vi "Vision Processing.vi"(4 "error in (no error)":errorcluster, 6 "CameraDevRef":T1) -> ()   [LabVIEW 2011]
uses:
  <vilib>/Rock Robotics/WPI/Camera/WPI_CameraDevRef.ctl
  Robot Global Data.vi
  <vilib>/vision/NI_Vision_Development_Module.lvlib
panel:
  in  "Scale":dbl=0.85
  in  "Minimum Power":dbl=0.2
  out "Aspect Ratio":dbl[](array[numeric])
  out "Offset":dbl
  in  "Max Distance for 1 hoop":dbl=8.0
  out "Raw Turret":dbl
  in  "Run Calculations":bool=TRUE
  out "Target X Coord":dbl
  out "Target Distance":dbl
  out "Target Y Coord":dbl
  out "Distance Array":dbl[](array[numeric])
  in  "Dead Band":dbl=0.1
  out "Number of Rectangles Visible":dbl
  out "Y Position Array":dbl[](array[numeric])
  out "X Position Array":dbl[](array[numeric])
  in  "View":bool
  out "Target Info":T2(array[cluster])
  in  "Area Size Limit":i32=444
  in  "Particle Count Limit":i32=8
  in  "Score Limits":T3={"Rect Coverage"=76.0, "Aspect Ratio"=40.0, "X Edge Strength"=40.0, "Y Edge Strength"=60.0}
  in  "Processing":enum32{"Color", "Intensity", "Intensity Open"}(tab)=enum."Intensity"
  in  "Luminance":i32=255
  in  "Saturation":i32=255
  in  "Hue":i32(knob)=65 scale=0.0..255.0
  in  "Margins":cluster{"Hue":i32, "Sat":i32, "Lum":i32}={"Hue"=20, "Sat"=27, "Lum"=30} {"Sat" scale=0.0..40.0; "Lum" scale=0.0..40.0; "Hue" scale=0.0..40.0}
  in  "Range":cluster{"Lower value":sgl, "Upper value":sgl}={"Lower value"=107.17391, "Upper value"=255.0} {"Lower value" scale=0.0..255.0; "Upper value" scale=0.0..255.0}
  in  "Range":cluster{"Lower value":sgl, "Upper value":sgl}={"Lower value"=123.804344, "Upper value"=255.0} {"Lower value" scale=0.0..255.0; "Upper value" scale=0.0..255.0}
  in  "View":bool
  out "Processed Image":T4(plugin-control)
  out "Original Image":T4(plugin-control)
  # "Instructions:\nProcessing the reflective tape that is illuminated by a ring light can be based\non color or light intensity.\nParticles within the image are scored by rectangle coverage, aspect ratio, and\nfor being hollow with a bold edge. A particle is considered a target if all scores\nare above the score limits. Particles can be annotated -- surrounded by\na rectangle and scores drawn to the left .\nTo control the number of particles being scored, use the count limit and the size\nlimit."
  # "(in)"
  # "To debug, Enable using the View button.\nFor color processing, you can click in the image to select the color for processing."
  # "Enable by clicking the View button.\nGreen scores are above the limit, orange are below. Inner/outer rect\nindicates all passed."
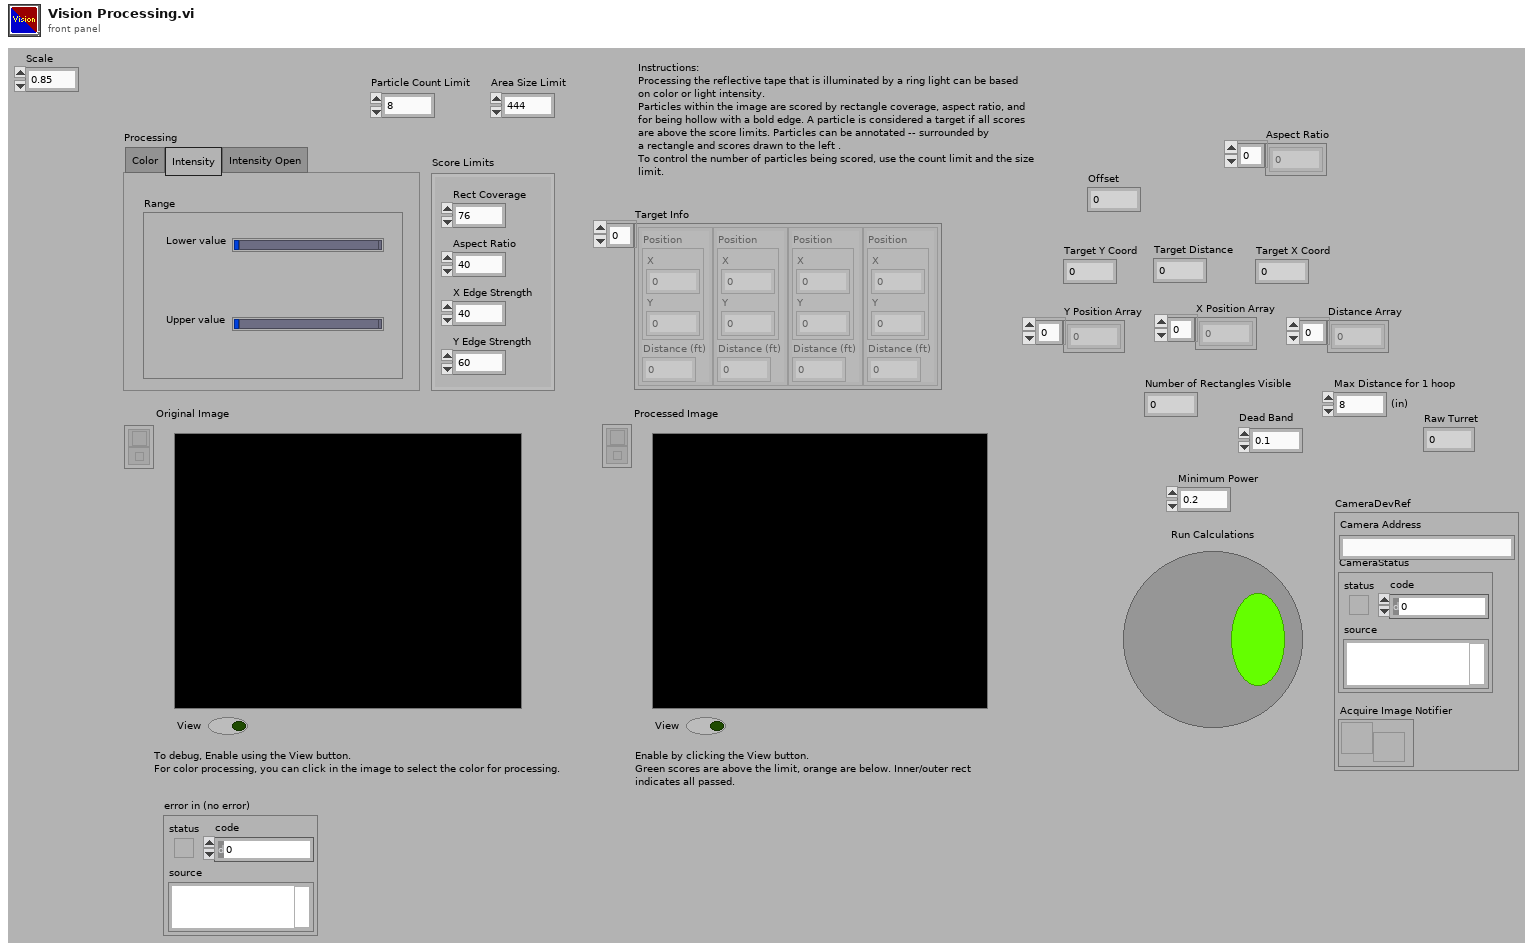
[diagram p1: front panel]
types:
  T1 = typedef "WPI_CameraDevRef.ctl" = cluster{"Camera Address":string, "CameraStatus":errorcluster, "Acquire Image Notifier":refnum<notifier>}
  T2 = cluster{"Position":cluster{"X":dbl, "Y":dbl}, "Distance (ft)":dbl}[]
  T3 = cluster{"Rect Coverage":dbl, "Aspect Ratio":dbl, "X Edge Strength":dbl, "Y Edge Strength":dbl}
  T4 = typedef "IMAQ Image.ctl" = refnum<image>
  T5 = typedef "Image Type" = u32
  T6 = enum32{"AutoM", "Close", "Dilate", "Erode", "Gradient", "Gradient out", "Gradient in", "Hit miss", "Open", "PClose", "POpen", "Thick", "Thin"}
  T7 = typedef "WPI_CameraImageSize.ctl" = enum16{"640x480", "320x240", "160x120"}
  T8 = cluster{"fps":i32, "compression":i32, "Image Size":T7}
  T9 = cluster{cluster{"Left":dbl, "Top":dbl, "Right":dbl, "Bottom":dbl}, dbl[]}[]
  T10 = cluster{"Left":dbl, "Top":dbl, "Right":dbl, "Bottom":dbl}
  T11 = cluster{"Target Center (-1 to 1)":cluster{"X":dbl, "Y":dbl}, "Distance (ft)":dbl}
  T12 = cluster{"Target Center (-1 to 1)":cluster{"X":dbl, "Y":dbl}, "Distance (ft)":dbl}[]
  T13 = typedef "WPI_JoystickDevRef.ctl" = cluster{"Device":T14}
  T14 = typedef "WPI_JoystickDeviceEnum.ctl" = enum16{"USB 1", "USB 2", "USB 3", "USB 4", "Kinect 1", "Kinect 2"}
  T15 = typedef "WPI_JoystickButtonState.ctl" = cluster{"Button 1":bool, "Button 2":bool, "Button 3":bool, "Button 4":bool, "Button 5":bool, "Button 6":bool, "Button 7":bool, "Button 8":bool, "Button 9":bool, "Button 10":bool, "Button 11":bool, "Button 12":bool}
  T16 = cluster{"axis 1 (x)":dbl, "axis 2 (y)":dbl, "axis 3 (throttle)":dbl, "axis 4":dbl, "axis 5":dbl, "axis 6":dbl}
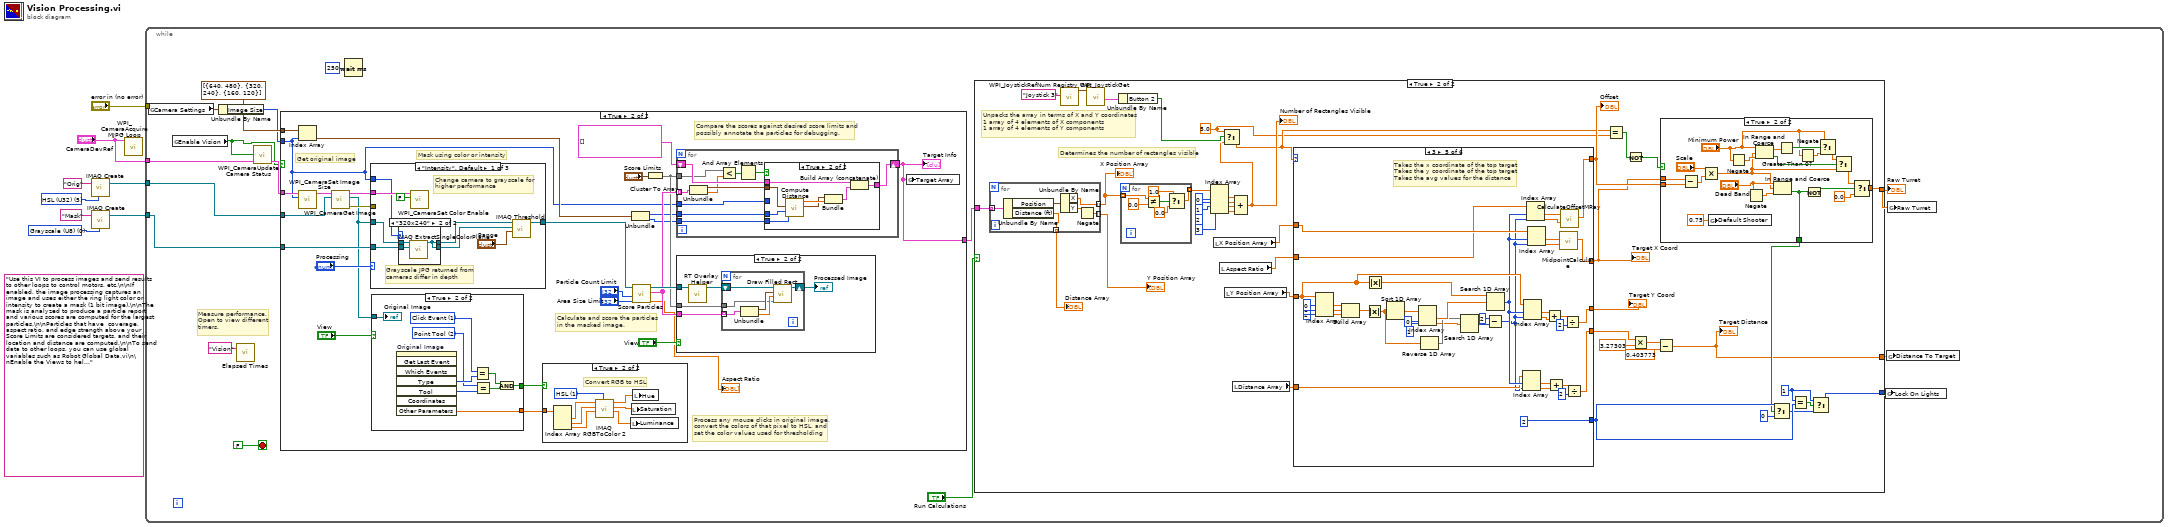
[diagram p0: block diagram]
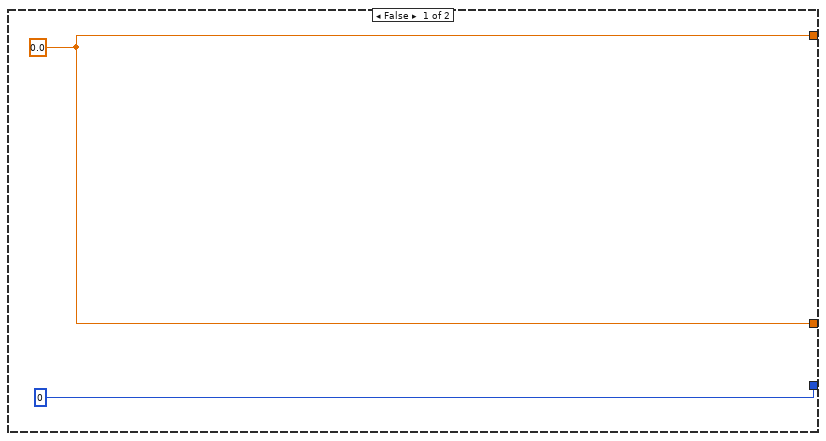
[diagram p2: hidden frame]
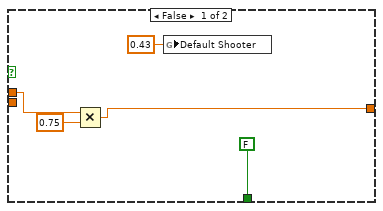
[diagram p3: hidden frame]
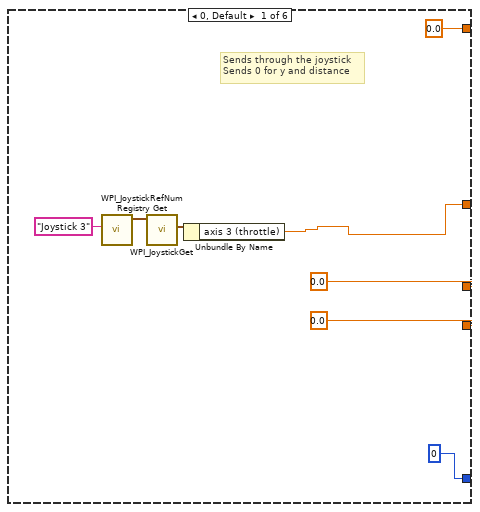
[diagram p4: hidden frame]
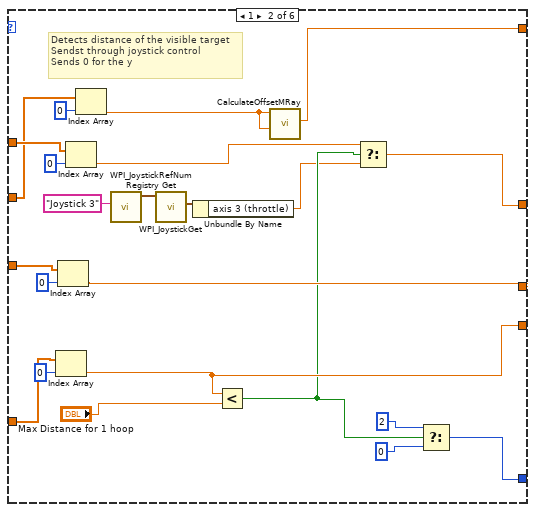
[diagram p5: hidden frame]
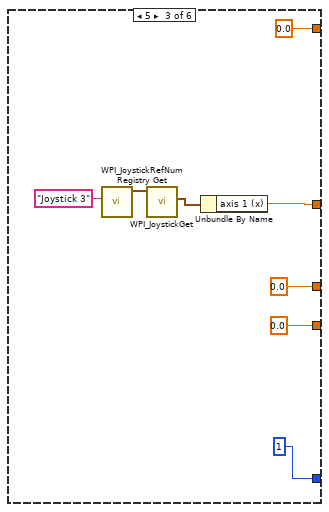
[diagram p6: hidden frame]
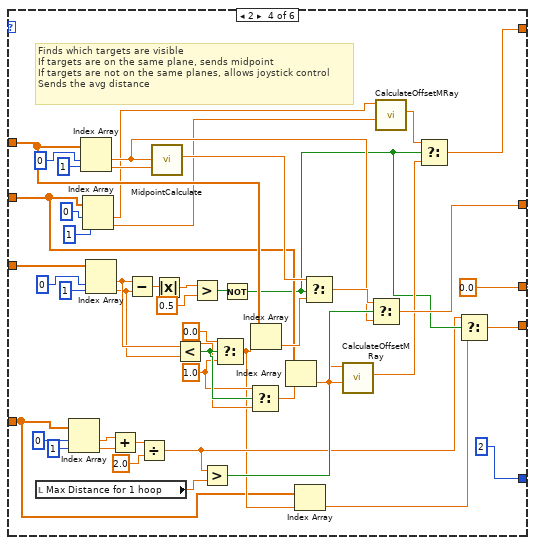
[diagram p7: hidden frame]
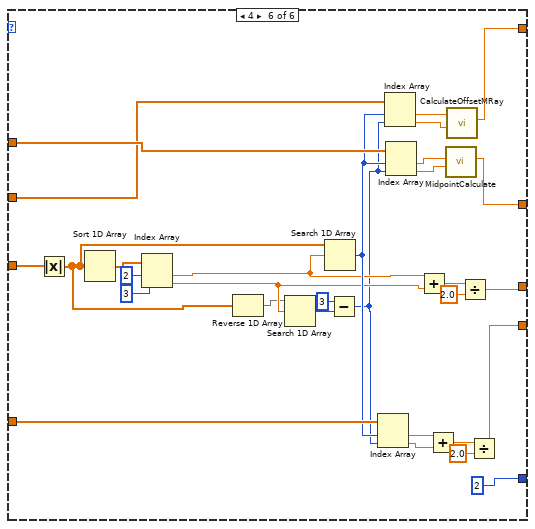
[diagram p8: hidden frame]
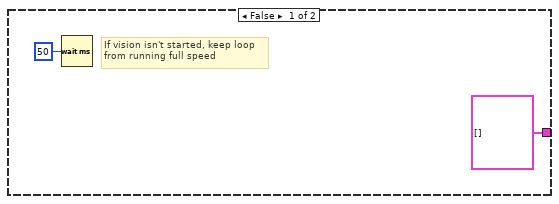
[diagram p9: hidden frame]
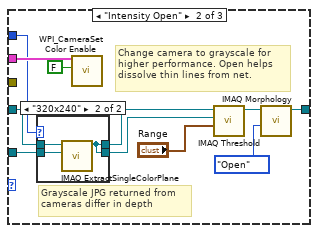
[diagram p12: hidden frame]
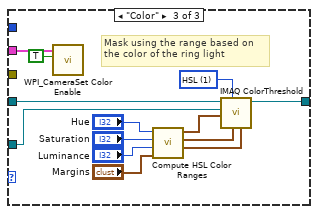
[diagram p14: hidden frame]
diagram:
  w3 = T5 0 items=["Grayscale (U8)", "Grayscale (I16)", "Grayscale (SGL)", "Complex (CSG)", "RGB (U32)", "HSL (U32)", "RGB (U64)", "Grayscale (U16)"] ("Image Type")
  (unwired) "Use this VI to process images and send results to other loops to control motors, etc.\n\nIf enabled, the image processing captures an image and uses either the ring light color or intensity to create a mask (1 bit image).\n\nThe mask is analyzed to produce a particle report and various scores are computed for the largest particles.\n\nParticles that have  coverage, aspect ratio, and edge strength above your Score Limits are considered targets, and their location and distance are computed.\n\nTo send data to other loops, you can use global variables such as Robot Global Data.vi\n\nEnable the Views to help debug color settings. Disable the View to speed up processing."
  w7 = T5 5 items=["Grayscale (U8)", "Grayscale (I16)", "Grayscale (SGL)", "Complex (CSG)", "RGB (U32)", "HSL (U32)", "RGB (U64)", "Grayscale (U16)"] ("Image Type")
  n1 = call "IMAQ Create"("Image Name"="Orig", "Image Type"=w7) -> ("New Image"=w6:T4)  [unwired: 2 in, 2 out]
  n2 = call "IMAQ Create"("Image Name"="Mask", "Image Type"=w3) -> ("New Image"=w1:T4)  [unwired: 2 in, 2 out]
  n3 = call <vilib>:"WPI_CameraAcquire MJPG Loop.vi"("CameraDevRef"="CameraDevRef") -> ()  [unwired: 11 in]
  n4 = while {
    tunnel: w6 -> [w23]
    tunnel: "CameraDevRef" -> [w22]
    tunnel: "error in (no error)" -> [_]
    tunnel: w1 -> [w18]
    stop <- FALSE stop-if-true
    # "Measure performance.\nOpen to view different\ntimers."
    n5 = global read "Robot Global Data.vi" "Camera Settings"() -> (w16:T8)
    n6 = global read "Robot Global Data.vi" "Enable Vision"() -> (w20:bool)
    n7 = Unbundle By Name(w16) -> ("Image Size"=w15:T7)
    n8 = call "Elapsed Times.vi"("Call Name"="Vision") -> ()  [unwired: 2 in, 1 out]
    n9 = call <vilib>:"WPI_CameraUpdate Camera Status.vi"("CameraDevRef In"=w22, "Enable Vision"=w20) -> ("CameraDevRef Out"=w21:T1)  [unwired: 3 in]
    n10 = case shown="True" w20 {
      tunnel: w23 -> [_ w281]
      tunnel: w21 -> [_ w277]
      tunnel: w18 -> [_ w268]
      tunnel: cluster{i32, i32}[] [{640, 480}, {320, 240}, {160, 120}] -> [_ w272]
      tunnel: w15 -> [_ w265]
      tunnel: [T2 [] w266] -> w14
      frame False {
        # "If vision isn't started, keep loop\nfrom running full speed"
        n11 = Wait (ms)(milliseconds to wait=u32 50) -> ()  [unwired: 1 out]
      }
      frame True {
        # "Compare the scores against desired score limits and\npossibly annotate the particles for debugging."
        # "Process any mouse clicks in original image,\nconvert the colors of that pixel to HSL, and\nset the color values used for thresholding"
        # "Calculate and score the particles\nin the masked image."
        # "Mask using color or intensity"
        # "Get original image"
        n12 = call <vilib>:"WPI_CameraSet Image Size.vi"("Image Size"=w265, "CameraDevRef"=w277) -> ("CameraDevRef Out"=w278:T1)  [unwired: 8 in, 1 out]
        n13 = Index Array(array=w272, index=w265) -> (element=w269:cluster{i32, i32})
        n14 = call <vilib>:"WPI_CameraGet Image.vi"("Image"=w281, "CameraDevRef"=w278) -> ("error out"=w279:errorcluster, "Image Out"=w267:T4, "CameraDevRef Out"=w280:T1)  [unwired: 7 in]
        n15 = case shown="\"Intensity\", Default" "Processing" {
          tunnel: w267 -> [w303 w315 w341]
          tunnel: [w306 w320 w340] -> w275
          tunnel: w280 -> [w304 w318 w331]
          tunnel: w279 -> [_ _ _]
          tunnel: w268 -> [w302 w316 w329]
          tunnel: w265 -> [w301 w317 _]
          frame "Intensity", Default {
            # "Grayscale JPG returned from\ncameras differ in depth"
            # "Change camera to grayscale for\nhigher performance"
            n16 = case shown="\"320x240\"" w301 {
              tunnel: w303 -> [w309 w312]
              tunnel: w302 -> [w308 w311]
              tunnel: [w309 w310] -> w300
              tunnel: [w308 w310] -> w299
              frame "640x480", Default {
              }
              frame "320x240" {
                n17 = call "IMAQ ExtractSingleColorPlane"("Image Dst"=w311, "Image Src"=w312) -> ("Image Dst Out"=w310:T4)  [unwired: 8 in, 1 out]
              }
            }
            n18 = call <vilib>:"WPI_CameraSet Color Enable.vi"("Color Enabled"=FALSE, "CameraDevRef"=w304) -> ()  [unwired: 8 in, 2 out]
            n19 = call "IMAQ Threshold"("Range"="Range", "Image Dst"=w299, "Image Src"=w300) -> ("Image Dst Out"=w306:T4)  [unwired: 3 in, 5 out]
          }
          frame "Intensity Open" {
            # "Grayscale JPG returned from\ncameras differ in depth"
            # "Change camera to grayscale for\nhigher performance. Open helps\ndissolve thin lines from net."
            n20 = case shown="\"320x240\"" w317 {
              tunnel: w315 -> [w325 w328]
              tunnel: w316 -> [w324 w327]
              tunnel: [w325 w326] -> w314
              tunnel: [w324 w326] -> w313
              frame "640x480", Default {
              }
              frame "320x240" {
                n21 = call "IMAQ ExtractSingleColorPlane"("Image Dst"=w327, "Image Src"=w328) -> ("Image Dst Out"=w326:T4)  [unwired: 8 in, 1 out]
              }
            }
            n22 = call <vilib>:"WPI_CameraSet Color Enable.vi"("Color Enabled"=FALSE, "CameraDevRef"=w318) -> ()  [unwired: 8 in, 2 out]
            n23 = call "IMAQ Threshold"("Range"="Range", "Image Dst"=w313, "Image Src"=w314) -> ("Image Dst Out"=w321:T4)  [unwired: 3 in, 5 out]
            n24 = call "IMAQ Morphology"("Operation"=T6."Open", "Image Src"=w321) -> ("Image Dst Out"=w320:T4)  [unwired: 8 in, 1 out]
          }
          frame "Color" {
            w339 = u16 1 items=["RGB", "HSL", "HSV", "HSI"] ("Color Mode")
            # "Mask using the range based on\nthe color of the ring light"
            n25 = call <vilib>:"WPI_CameraSet Color Enable.vi"("Color Enabled"=TRUE, "CameraDevRef"=w331) -> ()  [unwired: 8 in, 2 out]
            n26 = call "Compute HSL Color Ranges.vi"("Margins"="Margins", "Luminance"="Luminance", "Saturation"="Saturation", "Hue"="Hue") -> ("Lum Range"=w336:cluster{i32, i32}, "Sat Range"=w337:cluster{i32, i32}, "Hue Range"=w338:cluster{i32, i32})  [unwired: 5 in]
            n27 = call "IMAQ ColorThreshold"("Blue or Luma or Val or Inten Range"=w336, "Green or Sat Range"=w337, "Color Mode"=w339, "Red or Hue Range"=w338, "Image Dst"=w329, "Image Src"=w341) -> ("Image Dst Out"=w340:T4)  [unwired: 4 in, 1 out]
          }
        }
        n28 = case shown="True" "View" {
          tunnel: w267 -> [_ w361]
          tunnel: [_ w356] -> w274
          tunnel: [_ w353] -> w273
          frame False {
          }
          frame True {
            w354 = 2 items=["None", "Selection Tool", "Point Tool", "Line Tool", "Rectangle Tool", "Oval Tool", "Polygon Tool", "ClosedFreehandTool", "Annulus Tool", "Rotated Rectangle Tool", "Zoom Tool", "Pan Tool", "Polyline Tool", "Freehand Tool"] ("Tool")
            w355 = 1 items=["No Event"=0, "Click Event"=1, "Draw Event"=2, "Size Event"=4, "Scroll Event"=5, "Double Click Event"=8] ("Type")
            n29 = invoke on="Original Image" class="ImageControl" method="Get Last Event"() -> ("Type"=w357:i32, "Tool"=w360:i32, "Other Parameters"=w353:sgl[])  [unwired: 8 in, 5 out]
            n30 = Equal?(x=w355, y=w357) -> (x = y?=w358:bool)
            n31 = Equal?(x=w354, y=w360) -> (x = y?=w359:bool)
            n32 = And(x=w358, y=w359) -> (x .and. y?=w356:bool)
            "Original Image" <- w361
          }
        }
        n33 = case shown="True" w274 {
          tunnel: w273 -> [_ w298]
          frame False {
          }
          frame True {
            w297 = u16 1 items=["RGB", "HSL", "HSV", "HSI", "CIE L*a*b*", "CIE XYZ"] ("Color Mode")
            # "Convert RGB to HSL"
            n34 = Index Array(array=w298) -> (element #1=w296:sgl, element #2=w294:sgl, element #3=w292:sgl)  [unwired: 3 in]
            n35 = call "IMAQ RGBToColor 2"("Color Mode"=w297, "Blue value"=w292, "Green value"=w294, "Red value"=w296) -> ("Blue or Luma or Val or Inten or Z or b*value"=w291:dbl, "Green or Sat or Y or a* value"=w293:dbl, "Red or Hue or X or L* value"=w295:dbl)  [unwired: 4 in, 1 out]
            n36 = local write "Luminance"(w291) -> ()
            n37 = local write "Saturation"(w293) -> ()
            n38 = local write "Hue"(w295) -> ()
          }
        }
        n39 = Unbundle(w269) -> (w271:i32, w270:i32)
        n40 = call "Score Particles.vi"("Area Size Limit"="Area Size Limit", "Particle Count Limit"="Particle Count Limit", "Image Refnum in"=w275) -> ("Aspect Ratio"=→"Aspect Ratio":dbl[], "Scored Particle Info"=w286:T9, "Image Refnum out"=w289:T4)  [unwired: 6 in]
        n41 = Cluster To Array(cluster="Score Limits") -> (array=w284:dbl[])
        n42 = for {
          shift-right: [w371] -> w266
          shift-left: T2 [] -> [w372]
          tunnel: w271 -> [w370]
          tunnel: w286 -> [w368] mode=indexing
          tunnel: w284 -> [w363]
          tunnel: w265 -> [w367]
          tunnel: w270 -> [w362]
          n43 = Unbundle(w368) -> (w369:T10, w364:dbl[])
          n44 = Less?(x=w363, y=w364) -> (x < y?=w366:bool[])
          n45 = And Array Elements(Boolean array=w366) -> (logical AND=w365:bool)
          n46 = case shown="True" w365 {
            tunnel: w372 -> [w373 w381]
            tunnel: [w373 w380] -> w371
            tunnel: w369 -> [_ w376]
            tunnel: w370 -> [_ w378]
            tunnel: w367 -> [_ _]
            tunnel: w362 -> [_ w375]
            frame False {
            }
            frame True {
              n47 = call "Compute Distance.vi"("Y Image Resolution"=w375, "X Image Resolution"=w378, "Bounding Box"=w376) -> ("Target Center (-1 to 1)"=w374:cluster{"X":dbl, "Y":dbl}, "Distance (ft)"=w377:dbl)  [unwired: 7 in]
              n48 = Bundle("Target Center (-1 to 1)"=w374, "Distance (ft)"=w377) -> (w379:T11)  [unwired: 1 in]
              n49 = Build Array (concatenate)(w381, w379) -> (w380:T12)
            }
          }
        }
        "Target Info" <- w266
        n50 = case shown="True" "View" {
          tunnel: w289 -> [_ w343]
          tunnel: w286 -> [_ w345]
          tunnel: w284 -> [_ w344]
          frame False {
          }
          frame True {
            n51 = call "RT Overlay Helper.vi"("Refnum in"=w343) -> ("Refnum out"=w346:T4)  [unwired: 10 in]
            n52 = for {
              shift-right: [w351] -> w342
              shift-left: w346 -> [w352]
              tunnel: w345 -> [w348] mode=indexing
              tunnel: w344 -> [w347]
              n53 = Unbundle(w348) -> (w349:T10, w350:dbl[])
              n54 = call "Draw Filled Rect.vi"("Limits"=w347, "Scores"=w350, "Bounding Box"=w349, "image in"=w352) -> ("image out"=w351:T4)  [unwired: 7 in]
            }
            "Processed Image" <- w342
          }
        }
        n55 = global write "Robot Global Data.vi" "Target Array"(w266) -> ()
      }
    }
    n56 = Wait (ms)(milliseconds to wait=u32 250) -> ()  [unwired: 1 out]
    n57 = case shown="True" "Run Calculations" {
      tunnel: w14 -> [_ w52]
      tunnel: [w25 w37] -> w11
      tunnel: [0 ("f") w45] -> w10
      tunnel: [w25 w31] -> w9
      frame False {
        w25 = 0.0 ("f")
      }
      frame True {
        w46 = 1 ("y")
        w29 = 5.0 ("t")
        # "Determines the number of rectangles visible"
        # "Unpacks the array in terms of X and Y coordinates\n1 array of 4 elements of X components\n1 array of 4 elements of Y components"
        n58 = for {
          tunnel: [w259] -> w53 mode=indexing
          tunnel: [w260] -> w63 mode=indexing
          tunnel: w52 -> [w257] mode=indexing
          tunnel: [w256] -> w65 mode=indexing
          n59 = Unbundle By Name(w257) -> ("Position"=w261:cluster{"X":dbl, "Y":dbl}, "Distance (ft)"=w256:dbl)
          n60 = Unbundle By Name(w261) -> ("X"=w260:dbl, "Y"=w258:dbl)
          n61 = Negate(x=w258) -> (-x=w259:dbl)
        }
        "X Position Array" <- w63
        "Y Position Array" <- w53
        "Distance Array" <- w65
        n62 = call <vilib>:"WPI_JoystickRefNum Registry Get.vi"("refnum name"="Joystick 3") -> ("JoystickDevRef"=w51:T13)  [unwired: 9 in, 1 out]
        n63 = call <vilib>:"WPI_JoystickGet.vi"("JoystickDevRef"=w51) -> ("Buttons"=w49:T15)  [unwired: 4 in, 2 out]
        n64 = Unbundle By Name(w49) -> ("Button 2"=w48:bool)
        n65 = for {
          tunnel: w63 -> [w98] mode=indexing
          tunnel: [w94] -> w62 mode=indexing
          n66 = Not Equal?(x=w98, y=0.0) -> (x != y?=w97:bool)
          n67 = Select(t=1.0, s=w97, f=0.0) -> (s? t:f=w94:dbl)
        }
        n68 = Index Array(array=w62, index #1=0 ("index"), index #2=1 ("index"), index #3=2 ("index"), index #4=3 ("index")) -> (element #1=w60:dbl, element #2=w61:dbl, element #3=w59:dbl, element #4=w58:dbl)
        n69 = local read "X Position Array"() -> (w64:dbl[])
        n70 = local read "Aspect Ratio"() -> (w40:dbl[])
        n71 = local read "Y Position Array"() -> (w67:dbl[])
        n72 = local read "Distance Array"() -> (w68:dbl[])
        n73 = Compound Arithmetic op=ADD(w60, w61, w59, w58) -> (w41:dbl)
        "Number of Rectangles Visible" <- w41
        n74 = Select(t=w29, s=w48, f=w41) -> (s? t:f=w30:dbl)
        n75 = case shown="3" w30 {
          tunnel: w64 -> [_ w127 _ w153 w211 w251]
          tunnel: [w101 w121 w132 w162 w192 w247] -> w38
          tunnel: [0.0 ("X") w118 0.0 ("X") 0.0 ("X") w212 w246] -> w66
          tunnel: [0.0 ("X") w123 0.0 ("X") w144 w202 w241] -> w32
          tunnel: w67 -> [_ w119 _ w183 w207 w255]
          tunnel: w68 -> [_ w130 _ w140 w194 w250]
          tunnel: [0 w114 1 2 2 2] -> w44
          tunnel: [0.0 ("Offset") w111 0.0 ("Offset") w150 w199 w237] -> w39
          tunnel: w40 -> [_ w110 _ w145 w195 w233]
          frame 0, Default {
            # "Sends through the joystick\nSends 0 for y and distance"
            n76 = call <vilib>:"WPI_JoystickRefNum Registry Get.vi"("refnum name"="Joystick 3") -> ("JoystickDevRef"=w105:T13)  [unwired: 9 in, 1 out]
            n77 = call <vilib>:"WPI_JoystickGet.vi"("JoystickDevRef"=w105) -> ("Axes"=w103:T16)  [unwired: 4 in, 2 out]
            n78 = Unbundle By Name(w103) -> ("axis 3 (throttle)"=w101:dbl)
          }
          frame 1 {
            # "Detects distance of the visible target\nSendst through joystick control\nSends 0 for the y"
            n79 = Index Array(array=w130, index=0) -> (element=w123:dbl)
            n80 = Index Array(array=w119, index=0) -> (element=w118:dbl)
            n81 = Index Array(array=w127, index=0) -> (element=w112:dbl)
            n82 = Index Array(array=w110, index=0) -> (element=w108:dbl)
            n83 = call <vilib>:"WPI_JoystickRefNum Registry Get.vi"("refnum name"="Joystick 3") -> ("JoystickDevRef"=w126:T13)  [unwired: 9 in, 1 out]
            n84 = call <vilib>:"WPI_JoystickGet.vi"("JoystickDevRef"=w126) -> ("Axes"=w124:T16)  [unwired: 4 in, 2 out]
            n85 = Unbundle By Name(w124) -> ("axis 3 (throttle)"=w113:dbl)
            n86 = Less?(x=w123, y="Max Distance for 1 hoop") -> (x < y?=w116:bool)
            n87 = call "CalculateOffsetMRay.vi"("AR2"=w108, "AR1"=w108) -> ("Offset"=w111:dbl)  [unwired: 9 in]
            n88 = Select(t=w112, s=w116, f=w113) -> (s? t:f=w121:dbl)
            n89 = Select(t=2, s=w116, f=0) -> (s? t:f=w114:i32)
          }
          frame 5 {
            n90 = call <vilib>:"WPI_JoystickRefNum Registry Get.vi"("refnum name"="Joystick 3") -> ("JoystickDevRef"=w136:T13)  [unwired: 9 in, 1 out]
            n91 = call <vilib>:"WPI_JoystickGet.vi"("JoystickDevRef"=w136) -> ("Axes"=w134:T16)  [unwired: 4 in, 2 out]
            n92 = Unbundle By Name(w134) -> ("axis 1 (x)"=w132:dbl)
          }
          frame 2 {
            w156 = 1.0 ("f")
            w155 = 0.0 ("t")
            # "Finds which targets are visible\nIf targets are on the same plane, sends midpoint\nIf targets are not on the same planes, allows joystick control\nSends the avg distance"
            n93 = local read "Max Distance for 1 hoop"() -> (w164:dbl)
            n94 = Index Array(array=w140, index #1=0 ("index"), index #2=1 ("index")) -> (element #1=w171:dbl, element #2=w170:dbl)
            n95 = Index Array(array=w153, index #1=0 ("index"), index #2=1 ("index")) -> (element #1=w160:dbl, element #2=w159:dbl)
            n96 = Index Array(array=w145, index #1=0 ("index"), index #2=1 ("index")) -> (element #1=w147:dbl, element #2=w146:dbl)
            n97 = Index Array(array=w183, index #1=0 ("index"), index #2=1 ("index")) -> (element #1=w168:dbl, element #2=w167:dbl)
            n98 = Add(x=w171, y=w170) -> (x+y=w174:dbl)
            n99 = Subtract(x=w168, y=w167) -> (x-y=w180:dbl)
            n100 = Divide(x=w174, y=2.0) -> (x/y=w142:dbl)
            n101 = call "MidpointCalculate.vi"("X2"=w159, "X1"=w160) -> ("Midpoint"=w176:dbl)  [unwired: 9 in]
            n102 = Absolute Value(x=w180) -> (abs(x)=w179:dbl)
            n103 = Less?(x=w168, y=w167) -> (x < y?=w157:bool)
            n104 = Greater?(x=w179, y=0.5) -> (0:w177:bool)
            n105 = Greater?(x=w142, y=w164) -> (0:w163:bool)
            n106 = Select(t=w155, s=w157, f=w156) -> (s? t:f=w141:dbl)
            n107 = Not(x=w177) -> (.not. x?=w143:bool)
            n108 = Select(t=w156, s=w157, f=w155) -> (s? t:f=w154:dbl)
            n109 = Index Array(array=w153, index=w141) -> (element=w166:dbl)
            n110 = Index Array(array=w145, index=w154) -> (element=w152:dbl)
            n111 = Index Array(array=w140, index=w141) -> (element=w139:dbl)
            n112 = Select(t=w176, s=w143, f=w166) -> (s? t:f=w161:dbl)
            n113 = call "CalculateOffsetMRay.vi"("AR2"=w152, "AR1"=w152) -> ("Offset"=w151:dbl)  [unwired: 9 in]
            n114 = Select(t=w161, s=w163, f=w160) -> (s? t:f=w162:dbl)
            n115 = call "CalculateOffsetMRay.vi"("AR2"=w146, "AR1"=w147) -> ("Offset"=w158:dbl)  [unwired: 9 in]
            n116 = Select(t=w158, s=w143, f=w151) -> (s? t:f=w150:dbl)
            n117 = Select(t=w142, s=w143, f=w139) -> (s? t:f=w144:dbl)
          }
          frame 3 {
            # "Takes the x coordinate of the top target\nTakes the y coordinate of the top target\nTakes the avg values for the distance"
            n118 = Index Array(array=w207, index #1=0 ("index"), index #2=1 ("index"), index #3=2 ("index")) -> (element #1=w222:dbl, element #2=w221:dbl, element #3=w220:dbl)
            n119 = Build Array(w222, w221, w220) -> (w219:dbl[])
            n120 = Absolute Value(x=w219) -> (abs(x)=w190:dbl[])
            n121 = Absolute Value(x=w207) -> (abs(x)=w210:dbl[])
            n122 = Sort 1D Array(array=w190) -> (sorted array=w218:dbl[])
            n123 = Index Array(array=w218, index #1=0 ("index"), index #2=1 ("index")) -> (element #1=w215:dbl, element #2=w188:dbl)
            n124 = Reverse 1D Array(array=w190) -> (reversed array=w189:dbl[])
            n125 = Search 1D Array(1D array=w189, element=w188) -> (index of element=w191:i32)  [unwired: 1 in]
            n126 = Subtract(x=2, y=w191) -> (x-y=w186:i32)
            n127 = Search 1D Array(1D array=w210, element=w215) -> (index of element=w198:i32)  [unwired: 1 in]
            n128 = Index Array(array=w194, index #1=w198, index #2=w186) -> (element #1=w204:dbl, element #2=w203:dbl)
            n129 = Index Array(array=w207, index #1=w198, index #2=w186) -> (element #1=w209:dbl, element #2=w208:dbl)
            n130 = Index Array(array=w195, index #1=w198, index #2=w186) -> (element #1=w197:dbl, element #2=w196:dbl)
            n131 = Index Array(array=w211, index #1=w198, index #2=w186) -> (element #1=w193:dbl, element #2=w200:dbl)
            n132 = Add(x=w209, y=w208) -> (x+y=w214:dbl)
            n133 = Add(x=w204, y=w203) -> (x+y=w205:dbl)
            n134 = call "MidpointCalculate.vi"("X2"=w200, "X1"=w193) -> ("Midpoint"=w192:dbl)  [unwired: 9 in]
            n135 = call "CalculateOffsetMRay.vi"("AR2"=w196, "AR1"=w197) -> ("Offset"=w199:dbl)  [unwired: 9 in]
            n136 = Divide(x=w214, y=2) -> (x/y=w212:dbl)
            n137 = Divide(x=w205, y=2) -> (x/y=w202:dbl)
          }
          frame 4 {
            n138 = Absolute Value(x=w255) -> (abs(x)=w229:dbl[])
            n139 = Sort 1D Array(array=w229) -> (sorted array=w254:dbl[])
            n140 = Index Array(array=w254, index #1=2 ("index"), index #2=3 ("index")) -> (element #1=w232:dbl, element #2=w231:dbl)
            n141 = Reverse 1D Array(array=w229) -> (reversed array=w230:dbl[])
            n142 = Search 1D Array(1D array=w230, element=w231) -> (index of element=w228:i32)  [unwired: 1 in]
            n143 = Search 1D Array(1D array=w229, element=w232) -> (index of element=w236:i32)  [unwired: 1 in]
            n144 = Subtract(x=3, y=w228) -> (x-y=w227:i32)
            n145 = Index Array(array=w250, index #1=w236, index #2=w227) -> (element #1=w243:dbl, element #2=w242:dbl)
            n146 = Index Array(array=w233, index #1=w236, index #2=w227) -> (element #1=w234:dbl, element #2=w235:dbl)
            n147 = Index Array(array=w251, index #1=w236, index #2=w227) -> (element #1=w239:dbl, element #2=w238:dbl)
            n148 = Add(x=w232, y=w231) -> (x+y=w249:dbl)
            n149 = Add(x=w243, y=w242) -> (x+y=w244:dbl)
            n150 = call "MidpointCalculate.vi"("X2"=w238, "X1"=w239) -> ("Midpoint"=w247:dbl)  [unwired: 9 in]
            n151 = call "CalculateOffsetMRay.vi"("AR2"=w235, "AR1"=w234) -> ("Offset"=w237:dbl)  [unwired: 9 in]
            n152 = Divide(x=w249, y=2.0) -> (x/y=w246:dbl)
            n153 = Divide(x=w244, y=2.0) -> (x/y=w241:dbl)
          }
        }
        "Target Y Coord" <- w66
        "Target X Coord" <- w38
        "Offset" <- w39
        n154 = Equal?(x=w30, y=w29) -> (x = y?=w28:bool)
        n155 = Not(x=w28) -> (.not. x?=w27:bool)
        n156 = Multiply(x=w32, y=3.27303) -> (x*y=w34:dbl)
        n157 = Subtract(x=w34, y=0.403773) -> (x-y=w31:dbl)
        "Target Distance" <- w31
        n158 = case shown="True" w27 {
          tunnel: w39 -> [_ w92]
          tunnel: w38 -> [w72 w91]
          tunnel: [w70 w78] -> w37
          tunnel: [FALSE w76] -> w36
          frame False {
            n159 = Multiply(x=w72, y=0.75) -> (x*y=w70:dbl)
            n160 = global write "Robot Global Data.vi" "Default Shooter"(0.43 ("Right Limit")) -> ()
          }
          frame True {
            n161 = Subtract(x=w91, y=w92) -> (x-y=w89:dbl)
            n162 = Multiply(x="Scale", y=w89) -> (x*y=w80:dbl)
            n163 = global write "Robot Global Data.vi" "Default Shooter"(0.75 ("Right Limit")) -> ()
            n164 = Negate(x="Minimum Power") -> (-x=w87:dbl)
            n165 = Negate(x="Dead Band") -> (-x=w93:dbl)
            n166 = In Range and Coerce(upper limit="Minimum Power", x=w80, lower limit=w87) -> (coerced(x)=w83:dbl, In Range?=w84:bool)
            n167 = In Range and Coerce(upper limit="Dead Band", x=w80, lower limit=w93) -> (In Range?=w76:bool)  [unwired: 1 out]
            n168 = Greater Than 0?(x=w83) -> (x > 0?=w82:bool)
            n169 = Negate(x="Minimum Power") -> (-x=w79:dbl)
            n170 = Not(x=w76) -> (.not. x?=w77:bool)
            n171 = Select(t="Minimum Power", s=w82, f=w79) -> (s? t:f=w81:dbl)
            n172 = Select(t=w81, s=w84, f=w80) -> (s? t:f=w85:dbl)
            n173 = Select(t=w85, s=w77, f=0.0) -> (s? t:f=w78:dbl)
          }
        }
        n174 = Select(t=w44, s=w36, f=0) -> (s? t:f=w42:i32)
        n175 = Equal?(x=w46, y=w44) -> (x = y?=w47:bool)
        n176 = Select(t=w46, s=w47, f=w42) -> (s? t:f=w45:i32)
      }
    }
    "Raw Turret" <- w11
    n177 = global write "Robot Global Data.vi" "Lock On Lights"(w10) -> ()
    n178 = global write "Robot Global Data.vi" "Distance To Target"(w9) -> ()
    n179 = global write "Robot Global Data.vi" "Raw Turret"(w11) -> ()
  }
